vi "RSZVB Set Loss Reference Frequency.vi"(7 "Loss Reference Frequency (1.0e+9 Hz)":dbl=1000000000.0 format="%^.3e", 8 "error in (no error)":errorcluster {"code" format="%.0x"}, 9 "Port (1)":i32=1, 10 "Channel (1)":i32=1, 11 "VISA session":refnum<visa-resource-name>) -> (0 "error out":errorcluster {"code" format="%.0x"}, 3 "dup VISA session":refnum<visa-resource-name>)   [LabVIEW 2011]
doc: "This VI defines the reference frequency for the frequency-dependent part of the offset loss ([SENSe<Ch>:]CORRection:LOSS<port_no>:OFFSet).\n\nRemote-control command(s):\n[SENSe<Ch>:]CORRection:LOSS<port_no>:FREQuency <ref_frequency>"
uses:
  _utility/RSZVB Global Data.vi
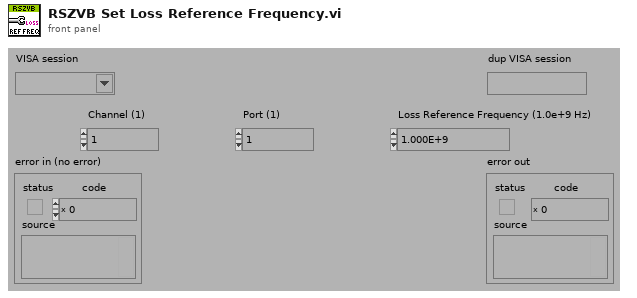
[diagram p1: front panel]
types:
  T1 = cluster{"Error Checking (T: On)":bool, "Installed Options":string[], "Data Valid?":bool, "Ports":i32, "Model":string[], "Option Checking (T: On)":bool}[]
  T2 = cluster{"Error Checking (T: On)":bool, "Installed Options":string[], "Data Valid?":bool, "Ports":i32, "Model":string[], "Option Checking (T: On)":bool}
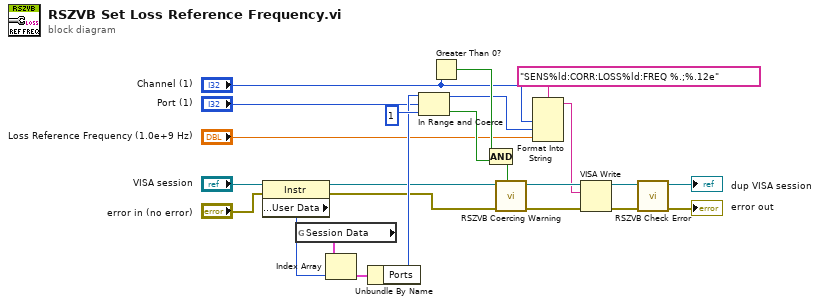
[diagram p0: block diagram]
diagram:
  n1 = property class="Instr"(reference="VISA session", error in="error in (no error)") -> (reference out=w10:refnum<visa-resource-name>, error out=w11:errorcluster, "General Settings:User Data"=w14:u32)
  n2 = global read "RSZVB Global Data.vi" "Session Data"() -> (w15:T1)
  n3 = Index Array(array=w15, index=w14) -> (element=w16:T2)
  n4 = Unbundle By Name(w16) -> ("Ports"=w12:i32)
  n5 = In Range and Coerce(upper limit=w12, x="Port (1)", lower limit=1) -> (coerced(x)=w9:i32, In Range?=w8:bool)
  n6 = Greater Than 0?(x="Channel (1)") -> (x > 0?=w17:bool)
  n7 = Compound Arithmetic op=AND(w17, w8) -> (w19:bool)
  n8 = call "RSZVB Coercing Warning.vi"("In Range?"=w19, "error in (no error)"=w11, "VISA session"=w10) -> ("error out"=w22:errorcluster, "dup VISA session"=w23:refnum<visa-resource-name>)  [unwired: 7 in]
  n9 = Format Into String(format string="SENS%ld:CORR:LOSS%ld:FREQ %.;%.12e", "Channel (1)", w9, "Loss Reference Frequency (1.0e+9 Hz)") -> (resulting string=w18:string)  [unwired: 2 in, 1 out]
  n10 = VISA Write(VISA resource name=w23, write buffer=w18, error in (no error)=w22) -> (VISA resource name out=w20:refnum<visa-resource-name>, error out=w21:errorcluster)  [unwired: 1 out]
  n11 = call "RSZVB Check Error.vi"("error in (no error)"=w21, "VISA session"=w20) -> ("error out"=→"error out":errorcluster, "dup VISA session"=→"dup VISA session":refnum<visa-resource-name>)  [unwired: 8 in]
